vi "File List Set Current File.vi"(9 "File":path, 10 "File index":i32, 11 "File List in":refnum<class "File List.lvclass">) -> (1 "Current file out":path, 2 "Current file index out":i32, 3 "File List out":refnum<class "File List.lvclass">)   [LabVIEW 2014, in "COSYLib.lvlib" / "File List.lvclass"]
doc: "Sets the currently active file.\nIf you wire a filename, that particular file is activated (if it is part of the list).\nElse, you can wire a File Index. This index is automatically coerced if necessary."
uses:
  File List.lvclass
  File List.lvclass/File List.ctl
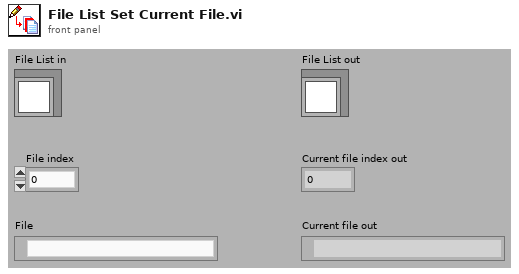
[diagram p1: front panel]
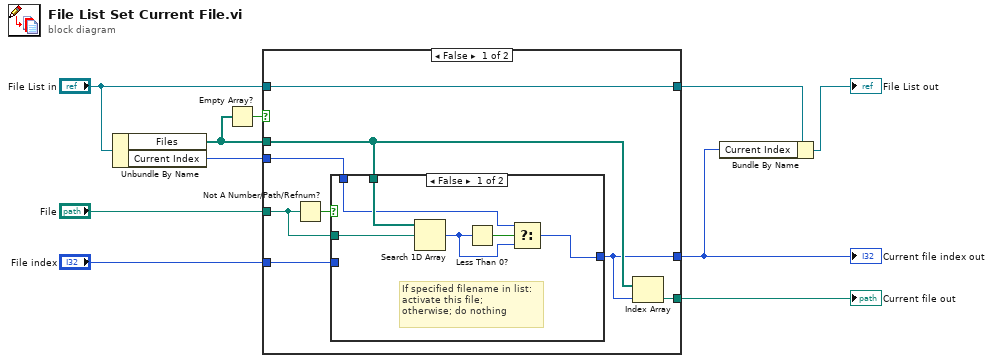
[diagram p0: block diagram]
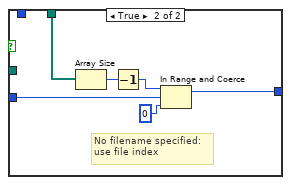
[diagram p2: hidden frame]
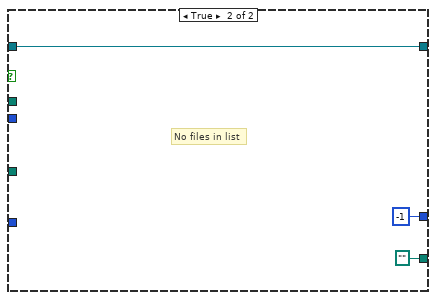
[diagram p3: hidden frame]
diagram:
  n1 = Unbundle By Name("File List in") -> ("Files"=w6:path[], "Current Index"=w8:i32)
  n2 = Empty Array?(array=w6) -> (empty?=w5:bool)
  n3 = case shown="False" w5 {
    tunnel: "File index" -> [w18 _]
    tunnel: w6 -> [w13 _]
    tunnel: "File" -> [w15 _]
    tunnel: w8 -> [w17 _]
    tunnel: [w11 -1 ("lower limit")] -> w7
    tunnel: "File List in" -> [w16 w31]
    tunnel: [w12 path ""] -> w3
    tunnel: [w16 w31] -> w2
    frame False {
      n4 = Not A Number/Path/Refnum?(number/path/refnum=w15) -> (NaN/Path/Refnum?=w14:bool)
      n5 = case shown="False" w14 {
        tunnel: w18 -> [_ w30]
        tunnel: [w20 w28] -> w11
        tunnel: w13 -> [w24 w26]
        tunnel: w15 -> [w23 _]
        tunnel: w17 -> [w21 _]
        frame False {
          # "If specified filename in list:\nactivate this file;\notherwise; do nothing"
          n6 = Search 1D Array(1D array=w24, element=w23) -> (index of element=w19:i32)  [unwired: 1 in]
          n7 = Less Than 0?(x=w19) -> (x < 0?=w22:bool)
          n8 = Select(t=w21, s=w22, f=w19) -> (s? t:f=w20:i32)
        }
        frame True {
          # "No filename specified:\nuse file index"
          n9 = Array Size(array=w26) -> (size(s)=w25:i32)
          n10 = Decrement(x=w25) -> (x-1=w27:i32)
          n11 = In Range and Coerce(upper limit=w27, x=w30, lower limit=0) -> (coerced(x)=w28:i32)  [unwired: 1 out]
        }
      }
      n12 = Index Array(array=w13, index=w11) -> (element=w12:path)
    }
    frame True {
      # "No files in list"
    }
  }
  "Current file index out" <- w7
  "Current file out" <- w3
  n13 = Bundle By Name(cluster=w2, "Current Index"=w7) -> (→"File List out":refnum<class "File List.lvclass">)
